vi "DisplayDataGlobal.vi"(7 "Action":T1, 11 "Set Value":dbl[][](array[numeric])) -> (3 "Value Out":dbl[][](array[numeric]))   [LabVIEW 2012]
uses:
  DisplayDataGlobalAction.ctl
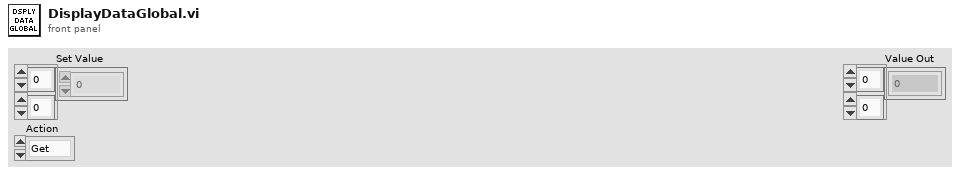
[diagram p1: front panel]
types:
  T1 = typedef "DisplayDataGlobalAction.ctl" = enum16{"Get", "Set"}
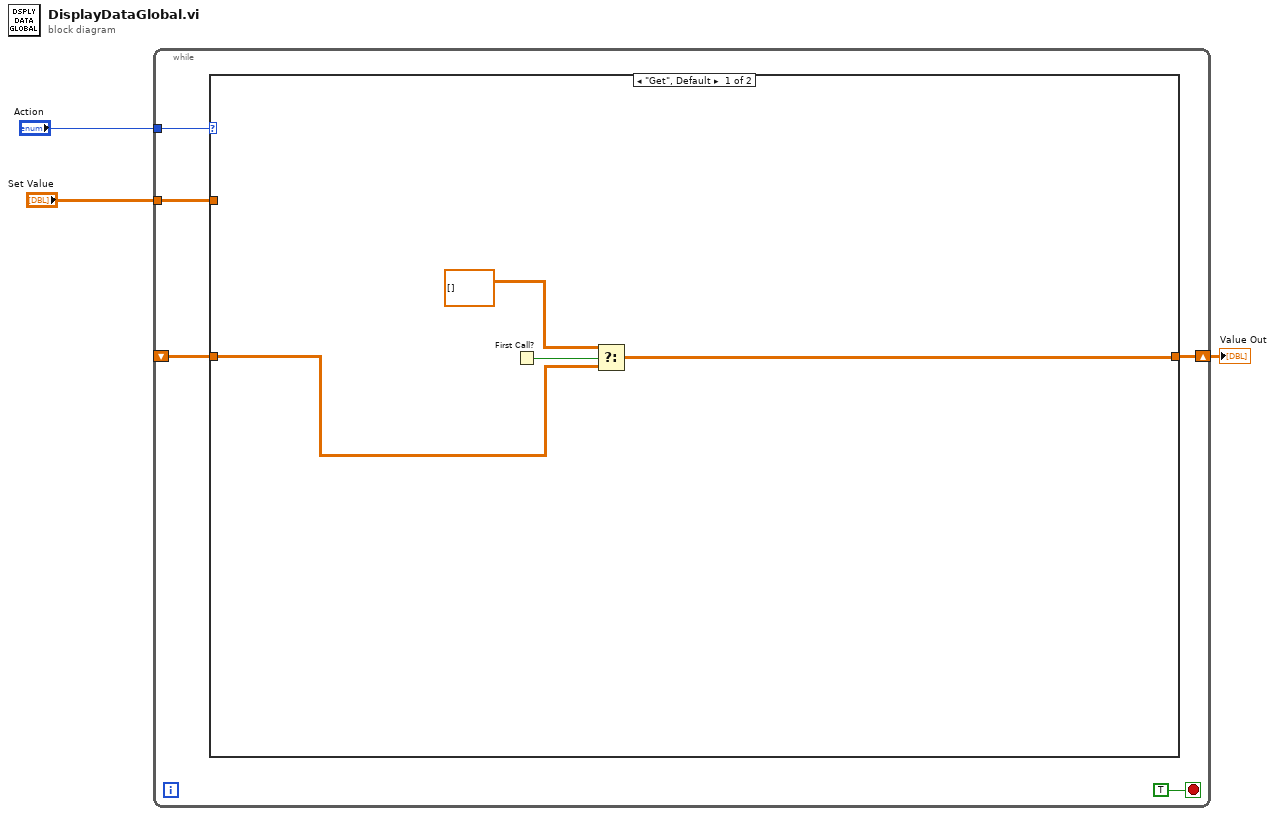
[diagram p0: block diagram]
diagram:
  n1 = while {
    tunnel: "Action" -> [w7]
    tunnel: "Set Value" -> [w6]
    shift-right: [w5] -> w1
    shift-left: _ -> [w4]
    stop <- TRUE stop-if-true
    n2 = case shown="\"Get\", Default" w7 {
      tunnel: w6 -> [_ w13]
      tunnel: [w11 w13] -> w5
      tunnel: w4 -> [w10 _]
      frame "Get", Default {
        n3 = First Call?() -> (First Call?: T/F=w12:bool)
        n4 = Select(t=dbl[][] [], s=w12, f=w10) -> (s? t:f=w11:dbl[][])
      }
      frame "Set" {
      }
    }
  }
  "Value Out" <- w1
